vi "DBPEN-LIN Balance Control.vi"() -> ()   [LabVIEW 2022 SP3]
uses:
  <vilib>/Simulation/Implementation/XNodeFramework/SimXNode/SimX.xnode
  <vilib>/Simulation/Implementation/Shared/SIMSCR Execution Mode.ctl
  <vilib>/Simulation/Scripting/Companion Diagram/SimConfigNode/_simSolvers.ctl
  <vilib>/Simulation/Scripting/Companion Diagram/SimConfigNode/SimParams.ctl
  <vilib>/Simulation/Scripting/Companion Diagram/SimConfigNode/SimDog.xnode
  <vilib>/Simulation/ContinuousLinear/Implementation/NILVSim Transfer Function.llb/SIM Transfer Function (SISO).vi
  <vilib>/Simulation/SignalArithmetic/Implementation/NILVSim Gain.llb/SIM Gain (scalar).vi
  <vilib>/Quanser/Rapid Control Prototyping Toolkit/hardware/HIL Immediate IO/CL HIL Write.vi
  <vilib>/Quanser/Rapid Control Prototyping Toolkit/hardware/HIL Immediate IO/CL HIL Read.vi
  <vilib>/Quanser/Rapid Control Prototyping Toolkit/hardware/HIL Immediate IO/_TypeSpecific/CL HIL Read Encoder (Vector).vi
  <vilib>/Simulation/DataSources/Implementation/NILVSim Signal Generator.llb/SIM Signal Generator (scalar).vi
  <vilib>/Simulation/SignalArithmetic/Implementation/NILVSim Gain.llb/SIM Gain (vector).vi
  <vilib>/Simulation/Utility/Implementation/SIM Halt.vi
  <vilib>/Simulation/SignalArithmetic/Implementation/NILVSim Gain.llb/SIM Gain (vector,MatrixGain).vi
  <vilib>/Simulation/ContinuousLinear/Implementation/NILVSim Integrator new.llb/SIM Integrator (scalar).vi
  <vilib>/Quanser/Rapid Control Prototyping Toolkit/hardware/HIL Immediate IO/_TypeSpecific/CL HIL Write Analog (Scalar).vi
  <vilib>/Simulation/Nonlinear/Implementation/NILVSim Saturation.llb/SIM Saturation (scalar).vi
panel:
  in  "Setpoint (mm)":dbl
  out "In Range?":bool=TRUE
  out "Short Pendulum Angle (deg)":dbl(graph)
  out "Medium Pendulum Angle (deg)":dbl(graph)
  out "Motor Voltage (V)":dbl(graph)
  in  "Gain":dbl[][](array[numeric])=[[42.329, -180.909, -417.766, 31.06, -48.496, -43.227, 10.0]] format="%.2f"
  out "IP02 Cart Position (mm)":cluster{"output":dbl, "output":dbl}(graph)
  in  "Stop Button":bool
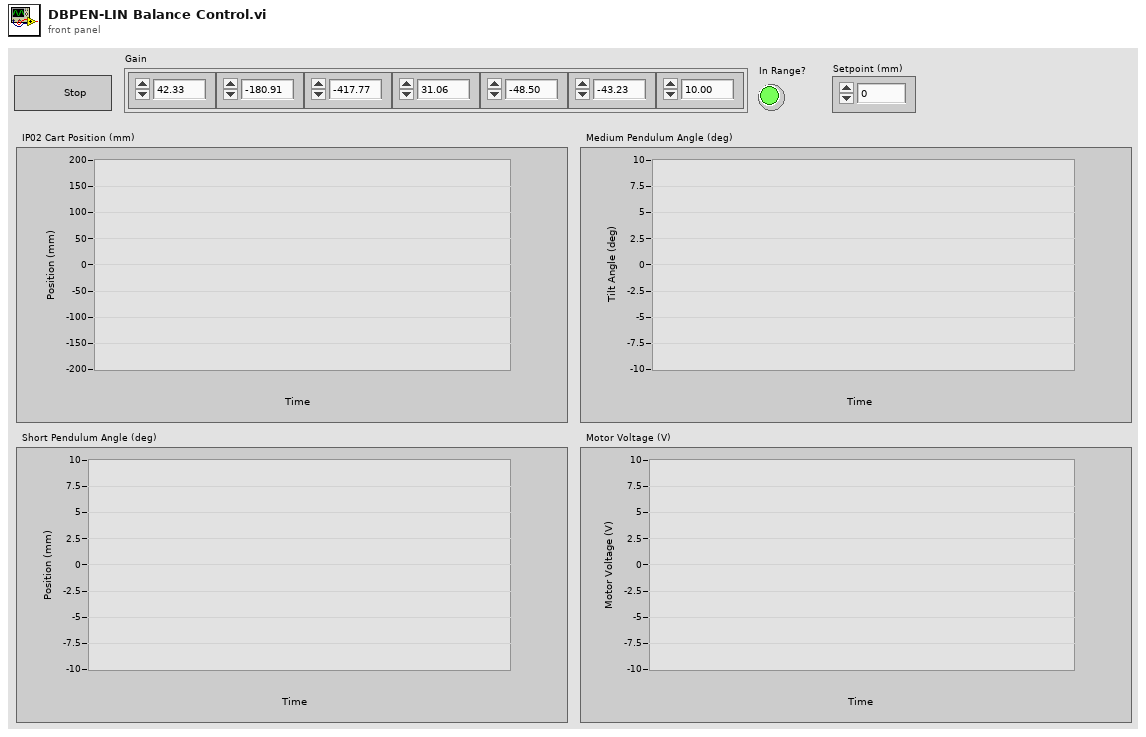
[diagram p1: front panel]
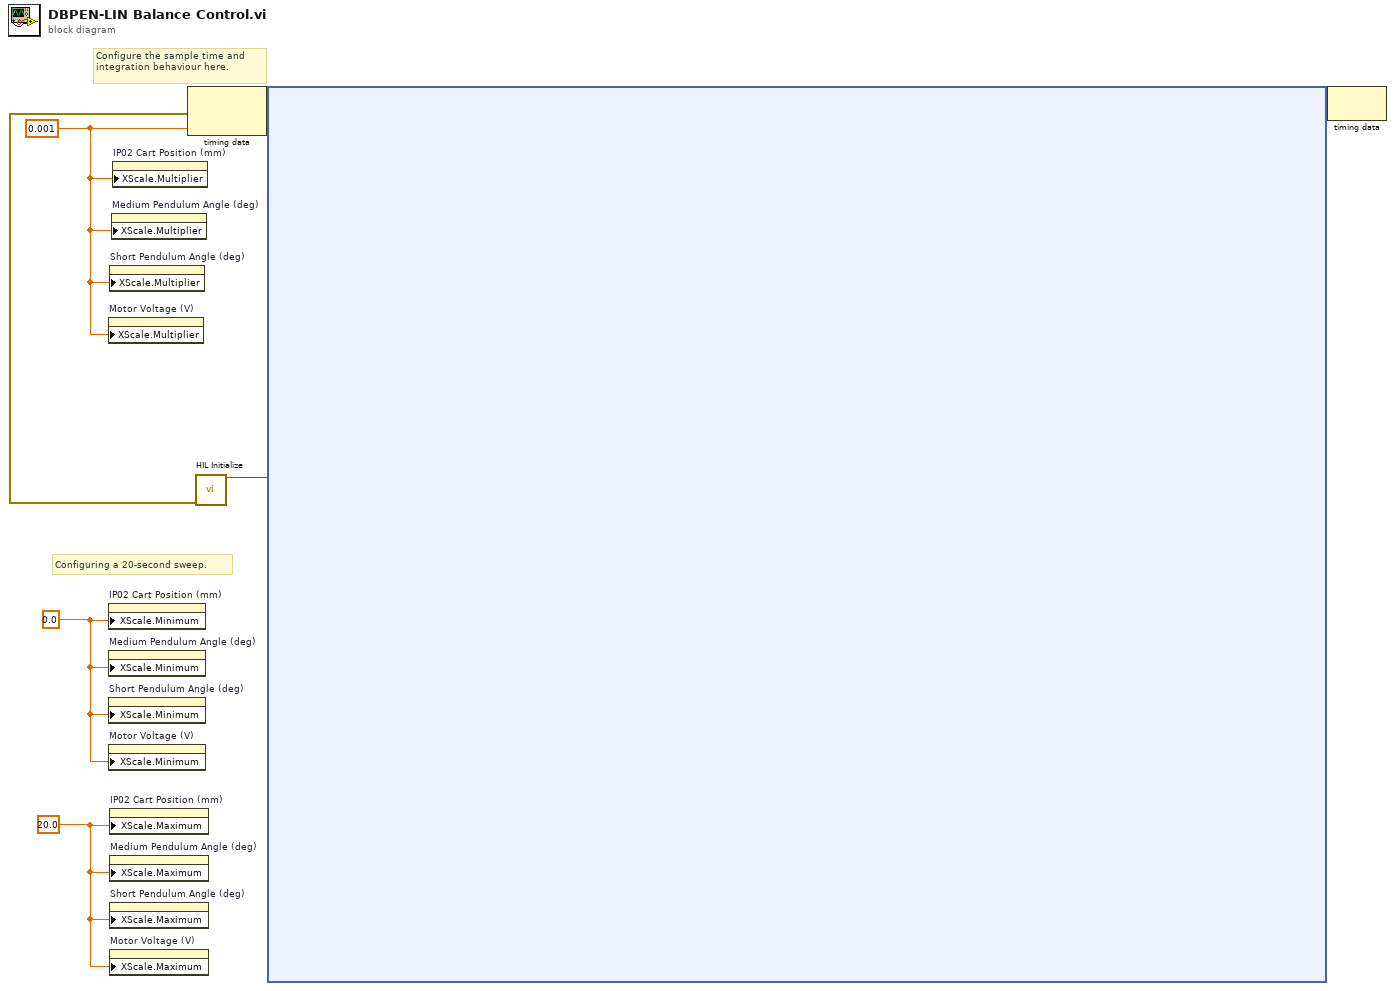
[diagram p0: block diagram]
diagram:
  w2 = 0.001 ("Step Size (s)")
  w4 = 0.0 ("X Scale.Range:Minimum")
  w3 = 20.0 ("X Scale.Range:Maximum")
  # "Configure the sample time and integration behaviour here."
  # "Configuring a 20-second sweep."
  n1 = property on="Motor Voltage (V)" class="WFChart (strict)"("XScale.Multiplier"=w2) -> ()  [unwired: 2 in, 2 out]
  n2 = property on="IP02 Cart Position (mm)" class="WFChart (strict)"("XScale.Minimum"=w4) -> ()  [unwired: 2 in, 2 out]
  n3 = property on="Medium Pendulum Angle (deg)" class="WFChart (strict)"("XScale.Minimum"=w4) -> ()  [unwired: 2 in, 2 out]
  n4 = property on="Short Pendulum Angle (deg)" class="WFChart (strict)"("XScale.Minimum"=w4) -> ()  [unwired: 2 in, 2 out]
  n5 = property on="Motor Voltage (V)" class="WFChart (strict)"("XScale.Minimum"=w4) -> ()  [unwired: 2 in, 2 out]
  n6 = property on="Short Pendulum Angle (deg)" class="WFChart (strict)"("XScale.Multiplier"=w2) -> ()  [unwired: 2 in, 2 out]
  n7 = property on="IP02 Cart Position (mm)" class="WFChart (strict)"("XScale.Maximum"=w3) -> ()  [unwired: 2 in, 2 out]
  n8 = property on="Medium Pendulum Angle (deg)" class="WFChart (strict)"("XScale.Maximum"=w3) -> ()  [unwired: 2 in, 2 out]
  n9 = property on="Short Pendulum Angle (deg)" class="WFChart (strict)"("XScale.Maximum"=w3) -> ()  [unwired: 2 in, 2 out]
  n10 = property on="Motor Voltage (V)" class="WFChart (strict)"("XScale.Maximum"=w3) -> ()  [unwired: 2 in, 2 out]
  n11 = property on="Medium Pendulum Angle (deg)" class="WFChart (strict)"("XScale.Multiplier"=w2) -> ()  [unwired: 2 in, 2 out]
  n12 = property on="IP02 Cart Position (mm)" class="WFChart (strict)"("XScale.Multiplier"=w2) -> ()  [unwired: 2 in, 2 out]
  n13 = call "HIL Initialize"() -> ("board out"=w5:refnum<class "HIL Board.lvclass">, "error out"=w1:errorcluster)  [unwired: 14 in]
  n14 = node-c288(w1, w2) -> (w7:variant)
  n15 = node-c254 ("Control & Simulation Loop")(w7, w5) -> (w6:variant)
  n16 = node-c288(w6) -> ()  [unwired: 1 out]
